vi "cqtdds_setSweep.vi"(8 "error in (no error)":errorcluster, 11 "input":T1={"Channel"=0, "AmplitudeScaleFactor"=683, "StartFrequency"=5000000.0, "StopFrequency"=30000000.0, "Rate"=3333000.0} {"Rate" format="%^#_6g"; "StopFrequency" format="%^#_6g"; "StartFrequency" format="%^#_6g"}) -> (0 "error out":errorcluster, 3 "Output":string="Rate = 3.333120248 MHz/s\r\nTotal Time = 7.500479 s")   [LabVIEW 2011]
uses:
  C:/Users/Administrator/Desktop/Crete/DDS/DDS-Control-a8929c3/CQTAD9958/bin/Debug/CQTAD9958.dll
  DDS-Control-a8929c3/CQTAD9958/bin/Debug/CQTAD9958.dll
panel:
  # "MHz"
  # "MHz"
  # "MHz/s"
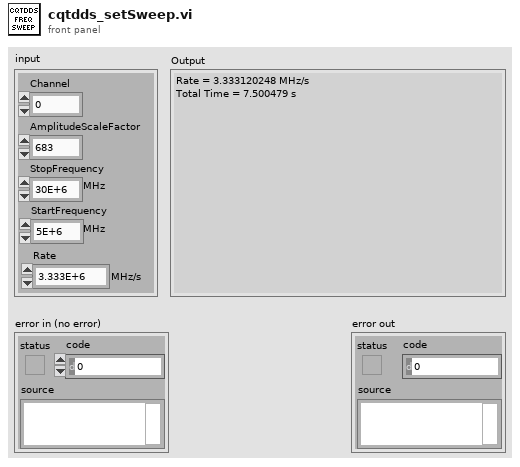
[diagram p1: front panel]
types:
  T1 = cluster{"Channel":i32, "AmplitudeScaleFactor":i32, "StartFrequency":dbl, "StopFrequency":dbl, "Rate":dbl}
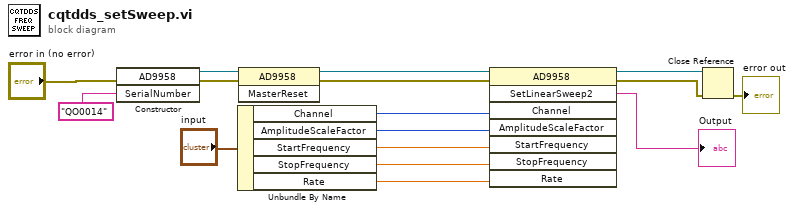
[diagram p0: block diagram]
diagram:
  n1 = constructor class="AD9958"(error in="error in (no error)", "SerialNumber"="QO0014") -> (reference out=w16:refnum<k24>, error out=w13:errorcluster)  [unwired: 2 in, 2 out]
  n2 = Unbundle By Name("input") -> ("Channel"=w7:i32, "AmplitudeScaleFactor"=w6:i32, "StartFrequency"=w5:dbl, "StopFrequency"=w4:dbl, "Rate"=w3:dbl)
  n3 = invoke class="AD9958" method="MasterReset"(reference=w16, error in=w13) -> (reference out=w14:refnum<k24>, error out=w12:errorcluster)  [unwired: 1 in, 1 out]
  n4 = invoke class="AD9958" method="SetLinearSweep2"(reference=w14, error in=w12, "Channel"=w7, "AmplitudeScaleFactor"=w6, "StartFrequency"=w5, "StopFrequency"=w4, "Rate"=w3) -> (reference out=w11:refnum<k24>, error out=w10:errorcluster, "SetLinearSweep2"=→"Output":string)  [unwired: 1 in, 5 out]
  n5 = Close Reference(reference=w11, error in (no error)=w10) -> (error out=→"error out":errorcluster)
